vi "I Doppler trigger signal using STFT.vi"() -> ()   [LabVIEW 2022 SP3]
doc: "Performs real-time Joint Time Frequency Analysis (JTFA) using Point By Point STFT. The signal is simulated by a sine wave plus Gaussian noise."
uses:
  <vilib>/measure/NI_MAPro.lvlib
  <vilib>/measure/mamon.llb/Waveform Peak Detection for N Chan.vi
  <resource>/objmgr/daqmx.rc
  <vilib>/gmath/NI_Gmath.lvlib
  <vilib>/DAQmx/read.llb/DAQmx Read (Analog 1D DBL 1Chan NSamp).vi
panel:
  out "Array 5":dbl[][](array[numeric])
  in  "DAQmx Task Name":refnum<k21>
  out "Waveform Graph 3":dbl[](graph)
  out "Waveform Graph 2":dbl[](graph)
  out "locations time 1":dbl[](array[numeric])
  out "locations time 0":dbl[](array[numeric])
  out "Locations":cluster{"Locations":dbl[]}[](array[cluster]) {"Locations" format="%.2p"}
  out "Amplitudes":cluster{"Amplitudes":dbl[]}[](array[cluster]) {"Amplitudes" format="%.2p"}
  out "# peaks found":i32[](array[numeric])
  out "Waveform Graph":dbl[][](graph)
  out "Array 3":dbl[][](array[numeric])
  out "DT":dbl
  out "Number of samples":dbl
  out "Number of cols (freq)":dbl
  out "Number of rows (time)":dbl
  out "Array 2":i32[](array[numeric])
  in  "time increment":i32=200
  out "Moving STFT":dbl[][](graph)
  in  "window length":i32=100 format="%0.0f"
  in  "stop":bool
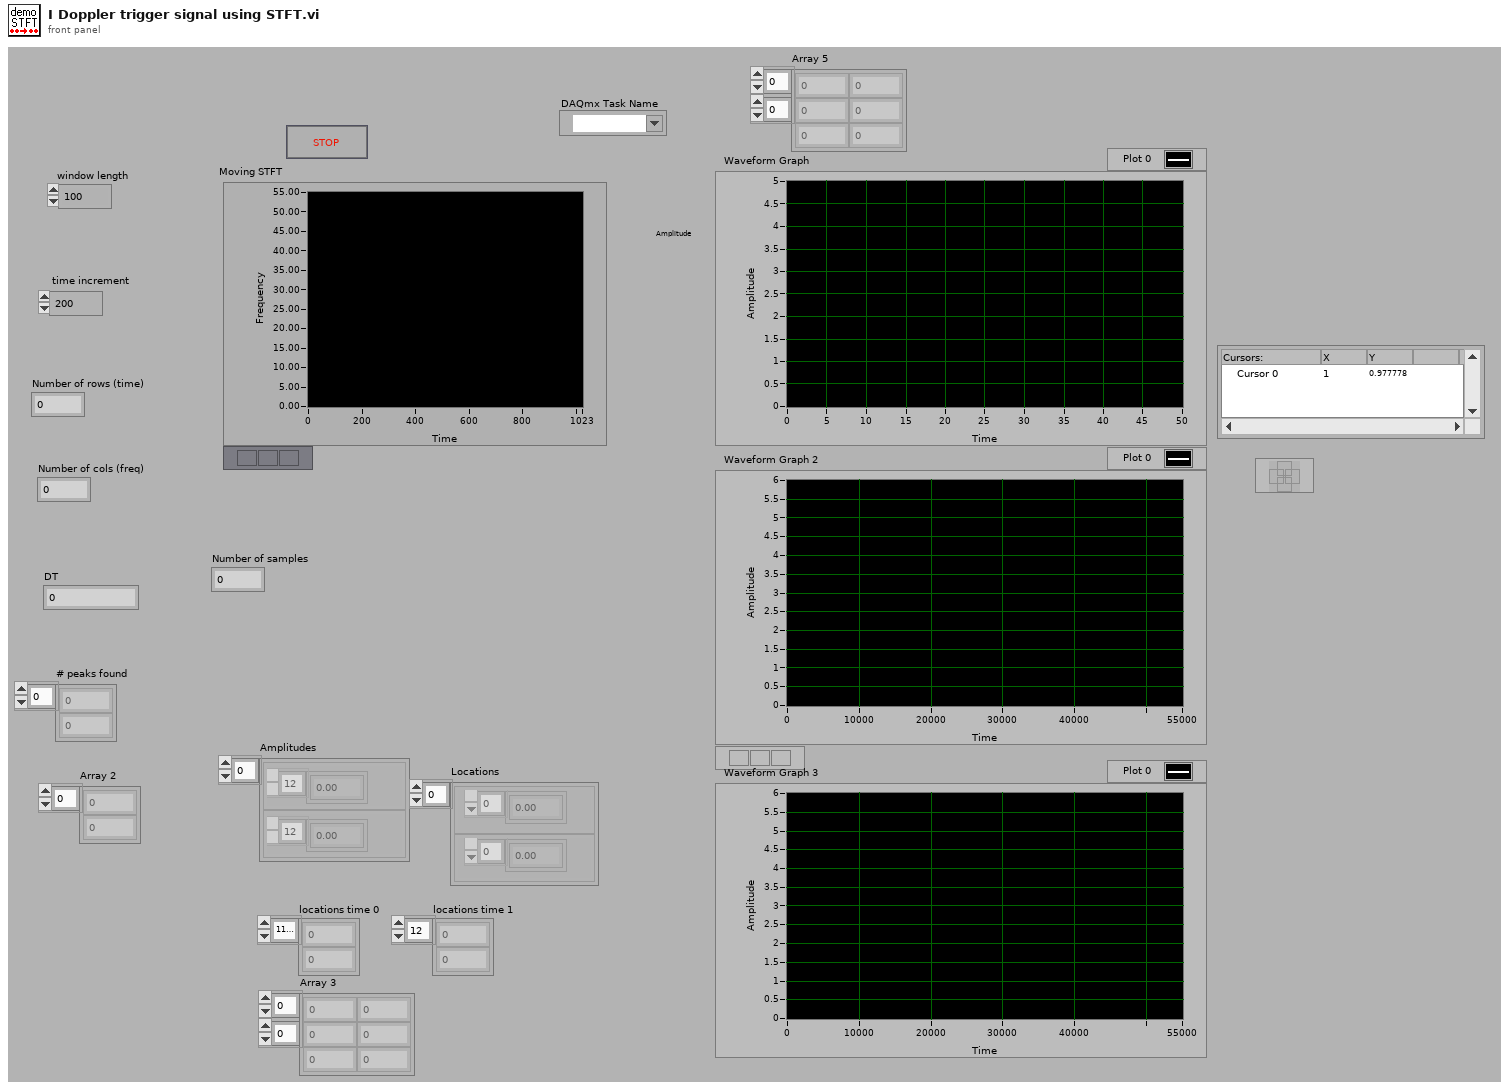
[diagram p1: front panel]
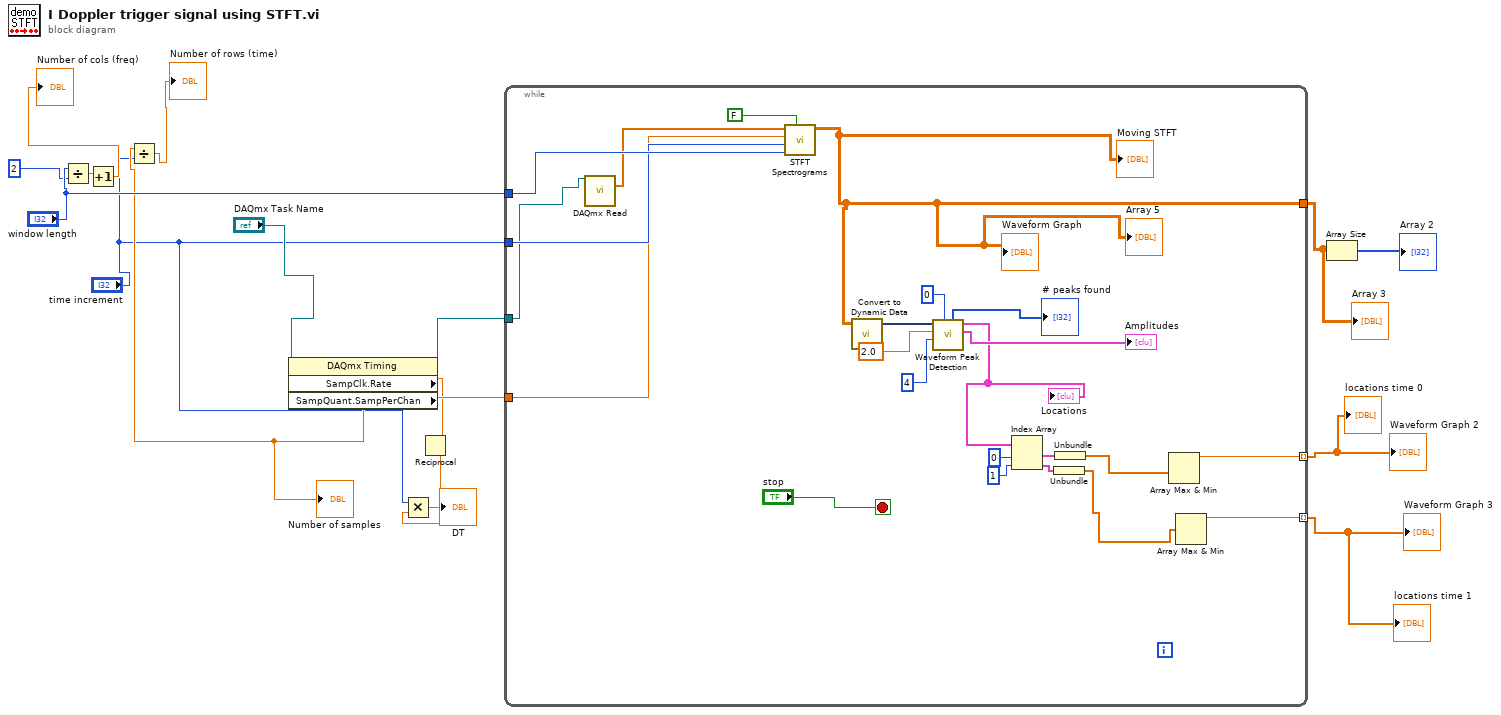
[diagram p0: block diagram]
diagram:
  n1 = Divide(x="window length", y=u32 2 ("milliseconds to wait")) -> (x/y=w16:dbl)
  n2 = Increment(x=w16) -> (x+1=→"Number of cols (freq)":dbl)
  n3 = property class="DAQmx Timing"(reference="DAQmx Task Name") -> (reference out=w6:refnum<k21>, "SampClk.Rate"=w2:dbl, "SampQuant.SampPerChan"=w5:dbl)  [unwired: 1 in, 1 out]
  "Number of samples" <- w5
  n4 = Divide(x=w5, y="time increment") -> (x/y=→"Number of rows (time)":dbl)
  n5 = Reciprocal(x=w2) -> (1/x=w1:dbl)
  n6 = Multiply(x="time increment", y=w1) -> (x*y=→"DT":dbl)
  n7 = while {
    tunnel: [w17] -> w12
    tunnel: [w25] -> w10 mode=indexing
    tunnel: [w24] -> w11 mode=indexing
    tunnel: "window length" -> [w22]
    tunnel: "time increment" -> [w21]
    tunnel: w6 -> [w18]
    tunnel: w5 -> [w19]
    stop <- "stop" stop-if-true
    n8 = call-poly <vilib>:"DAQmx Read.vi"("task/channels in"=w18) -> ("data"=w20:dbl[])  [unwired: 2 in, 12 out]
    n9 = call <vilib>:"STFT Spectrograms.vi"("energy conservation?"=FALSE, "window parameter"=w22, "window info"=w21, "time-freq sampling info"=w19, "X"=w20) -> ("STFT Spectrogram {X}"=w17:dbl[][])  [unwired: 5 in, 1 out]
    "Waveform Graph" <- w17
    "Moving STFT" <- w17
    "Array 5" <- w17
    n10 = call "Convert to Dynamic Data"("2D Array"=w17) -> ("Dynamic Data Type"=w38:dynamicdata)  [unwired: 3 out]
    n11 = call-poly <vilib>:"Waveform Peak Detection.vi"("peaks/valleys"=u32 0 ("milliseconds to wait"), "width"=u32 4 ("milliseconds to wait"), "threshold"=2.0 ("Y Scale.Range:Minimum"), "Signals In"=w38) -> ("Amplitudes"=→"Amplitudes":cluster{"Amplitudes":dbl[]}[], "Locations"=w32:cluster{"Locations":dbl[]}[], "# found"=→"# peaks found":i32[])  [unwired: 3 in, 2 out]
    "Locations" <- w32
    n12 = Index Array(array=w32, index #1=u32 0 ("milliseconds to wait"), index #2=u32 1 ("milliseconds to wait")) -> (element #1=w30:cluster{"Locations":dbl[]}, element #2=w28:cluster{"Locations":dbl[]})
    n13 = Unbundle(w28) -> ("Locations"=w26:dbl[])
    n14 = Unbundle(w30) -> ("Locations"=w27:dbl[])
    n15 = Array Max & Min(array=w27) -> (max value=w25:dbl)  [unwired: 3 out]
    n16 = Array Max & Min(array=w26) -> (max value=w24:dbl)  [unwired: 3 out]
  }
  "Array 3" <- w12
  "Waveform Graph 2" <- w10
  "Waveform Graph 3" <- w11
  "locations time 0" <- w10
  "locations time 1" <- w11
  n17 = Array Size(array=w12) -> (size(s)=→"Array 2":i32[])
